vi "XNET Signal to Frame.vi"(8 "error in (no error)":errorcluster, 9 "Data Array":dbl[](array[numeric]), 10 "Frame":string, 11 "CAN in":refnum<class "XNET_BS120x.lvclass">) -> (0 "error out":errorcluster, 2 "Data":refnum<class "XNET Data.lvclass">, 3 "CAN out":refnum<class "XNET_BS120x.lvclass">)   [LabVIEW 2021, in "BS120x Driver.lvlib" / "XNET_BS120x.lvclass"]
uses:
  XNET_BS120x.lvclass
  _Private/Data Classes/XNET Data Class/XNET Data.lvclass
  XNET_BS120x.lvclass/XNET_BS120x.ctl
  _Private/Data Classes/XNET Data Class/XNET Data.lvclass/XNET Data.ctl
  _Private/Data Classes/XNET Data Class/Write XNET Array.vi
  _Private/Data Classes/XNET Data Class/Write XNET Frame.vi
  <vilib>/xnet/xnet.llb/XNET Create Session (Conversion).vi
  <vilib>/xnet/xnet.llb/XNET Convert (Signal to Frame CAN).vi
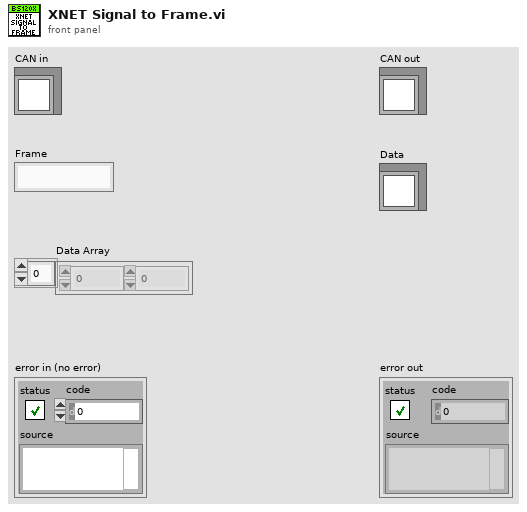
[diagram p1: front panel]
types:
  T1 = typedef "XNET Frame CAN.ctl" = cluster{"timestamp":timestamp, "payload":u8[], "identifier":u32, "type":T2, "extended?":bool, "echo?":bool}
  T2 = typedef "XNET Frame Type CAN.ctl" = u8
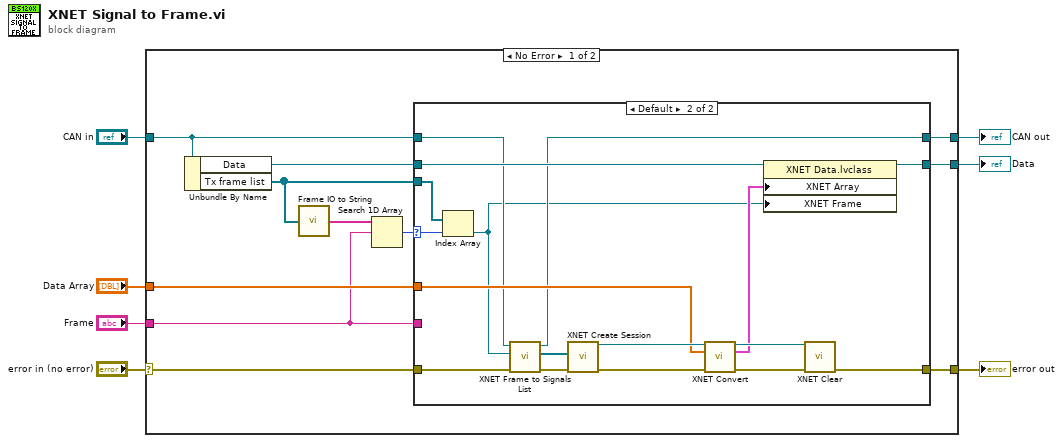
[diagram p0: block diagram]
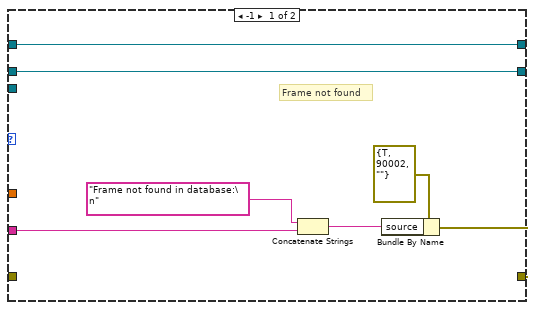
[diagram p2: hidden frame]
diagram:
  n1 = case shown="No Error" "error in (no error)" {
    selector: "error in (no error)" -> [w15 w44]
    tunnel: [w16 w44] -> w5
    tunnel: [w8 w43] -> w1
    tunnel: "CAN in" -> [w9 w43]
    tunnel: "Data Array" -> [w18 _]
    tunnel: [w17 _] -> w4
    tunnel: "Frame" -> [w12 _]
    frame No Error {
      n2 = Unbundle By Name(w9) -> ("Data"=w10:refnum<class "XNET Data.lvclass">, "Tx frame list"=w11:refnum<k21>[])
      n3 = call "Frame IO to String.vi"("Frame list"=w11) -> ("Frame list"=w13:string[])
      n4 = Search 1D Array(1D array=w13, element=w12) -> (index of element=w14:i32)  [unwired: 1 in]
      n5 = case shown="Default" w14 {
        selector: w14 -> [_ w33]
        tunnel: w10 -> [w25 w42]
        tunnel: w18 -> [_ w32]
        tunnel: [w25 w41] -> w17
        tunnel: [w20 w40] -> w16
        tunnel: w15 -> [_ w31]
        tunnel: w11 -> [_ w34]
        tunnel: w12 -> [w22 _]
        tunnel: w9 -> [w19 w28]
        tunnel: [w19 w27] -> w8
        frame -1 {
          # "Frame not found"
          n6 = Concatenate Strings("Frame not found in database:\n" ("source"), w22) -> (w21:string)
          n7 = Bundle By Name(cluster=errorcluster {"status"=TRUE, "code"=90002, "source"=""} ("error out"), "source"=w21) -> (w20:errorcluster)
        }
        frame Default {
          n8 = Index Array(array=w34, index=w33) -> (element=w26:refnum<k21>)
          n9 = call-dynamic "XNET Frame to Signals List.vi"("error in (no error)"=w31, "XNET Frame"=w26, "BS1200 in"=w28) -> ("error out"=w30:errorcluster, "Sorted XNET Signals"=w29:refnum<k21>[], "BS1200 out"=w27:refnum<class "XNET_BS120x.lvclass">)  [unwired: 6 in]
          n10 = call-poly <vilib>:"XNET Create Session.vi"("signal list"=w29, "error in (no error)"=w30) -> ("session out"=w39:refnum<k21>, "error out"=w37:errorcluster)  [unwired: 12 out]
          n11 = call-poly <vilib>:"XNET Convert.vi"("session in"=w39, "signal data"=w32, "error in (no error)"=w37) -> ("session out"=w38:refnum<k21>, "frame data"=w35:T1[], "error out"=w36:errorcluster)  [unwired: 10 out]
          n12 = property class="XNET Data.lvclass"(reference=w42, "XNET Array"=w35, "XNET Frame"=w26) -> (reference out=w41:refnum<class "XNET Data.lvclass">)  [unwired: 1 in, 1 out]
          n13 = call <vilib>:"XNET Clear.vi"("session in"=w38, "error in (no error)"=w36) -> ("error out"=w40:errorcluster)  [unwired: 13 in]
        }
      }
    }
    frame Error {
    }
  }
  "error out" <- w5
  "Data" <- w4
  "CAN out" <- w1
